vi "xiCam - StartAcquisition.vi"(8 "error in (no error)":errorcluster, 11 "xiCam In":refnum<k24>) -> (0 "error out":errorcluster, 3 "xiCam Out":refnum<k24>)   [LabVIEW 2016]
doc: "This function starts the data acquisition on the device.\n\n<b>void StartAcquisition()</b>"
uses:
  C:/Users/Ries Lab/Documents/Microscope Control from Sheng Account/Microscope-Control/Device Library/Cameras/Ximea/xiLIB_64bit/xiLIB/xiCamLib/API/x64/xiApi.NETX64.dll
  API/x64/xiApi.NETX64.dll
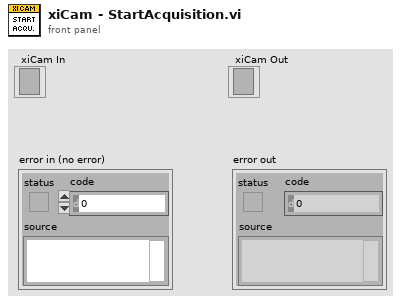
[diagram p1: front panel]
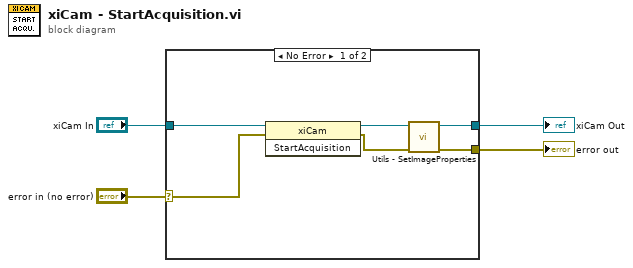
[diagram p0: block diagram]
diagram:
  n1 = case shown="No Error" "error in (no error)" {
    selector: "error in (no error)" -> [w9 w11]
    tunnel: "xiCam In" -> [w10 w12]
    tunnel: [w6 w12] -> w2
    tunnel: [w5 w11] -> w1
    frame No Error {
      n2 = invoke class="xiCam" method="StartAcquisition"(reference=w10, error in=w9) -> (reference out=w8:refnum<k24>, error out=w7:errorcluster)  [unwired: 1 in, 1 out]
      n3 = call "Utils - SetImageProperties.vi"("error in (no error)"=w7, "xiCam In"=w8) -> ("error out"=w5:errorcluster, "xiCam Out"=w6:refnum<k24>)  [unwired: 8 in]
    }
    frame Error {
    }
  }
  "error out" <- w1
  "xiCam Out" <- w2
